vi "channelGraphs.vi"(8 "error in (no error)":errorcluster, 10 "Clean+No Dups":string[][](array[string])) -> (0 "error out":errorcluster, 1 "Noisy Pixel List":i32[][](array[numeric]), 2 "Intensity Graph":u32[][](graph), 3 "Detector Surface":refnum<class "3D Plot Datatype.lvclass">[](xcontrol), 5 "Event Count Histogram":T1(graph))   [LabVIEW 2019]
uses:
  <vilib>/Analysis/NI_AALBase.lvlib
  <vilib>/Math Plots/3D Math Plots/3D Surface/3D Surface Datatype/3D Surface Datatype.lvclass
  <vilib>/Math Plots/3D Math Plots/3D Surface/3D Surface Datatype/Public/Plot Helper (Vector).vi
  <vilib>/Math Plots/3D Math Plots/3D Surface/3D Surface XCtrl/3D Surface.xctl
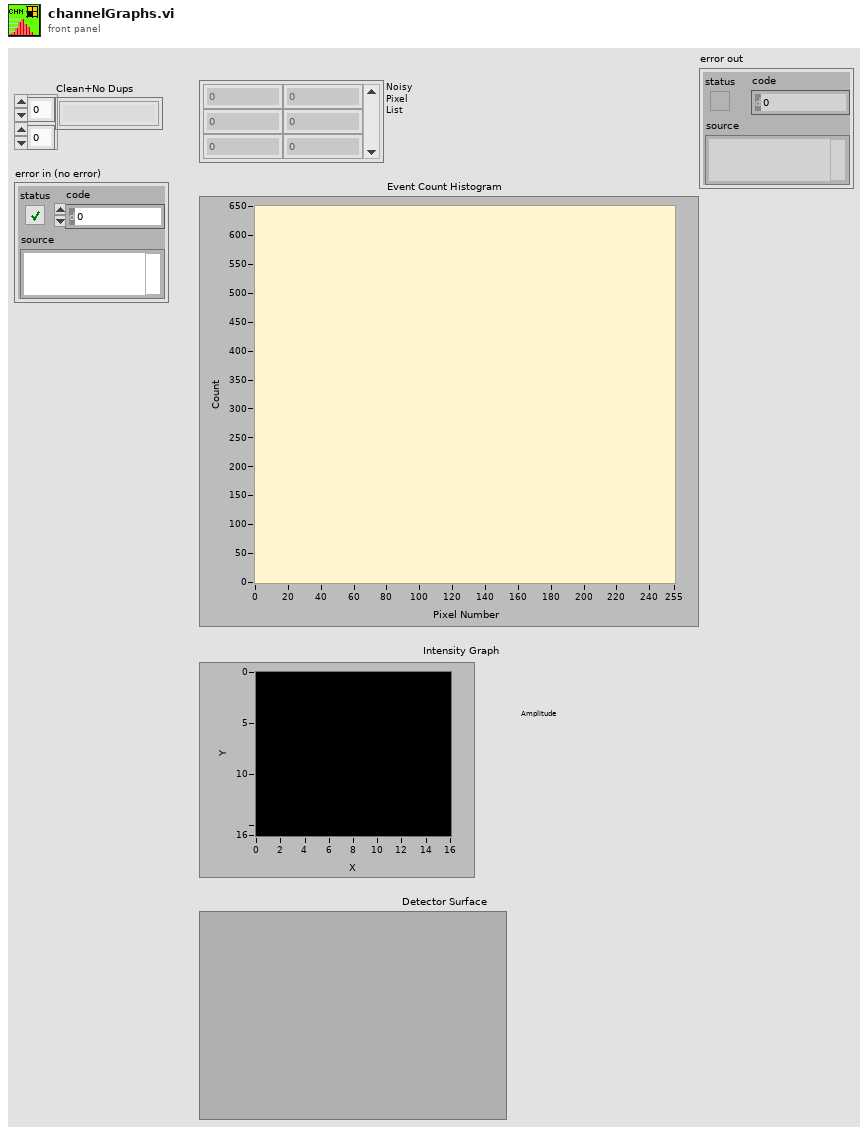
[diagram p1: front panel]
types:
  T1 = cluster{"X Values":dbl[], "Histogram: h(x)":i32[]}
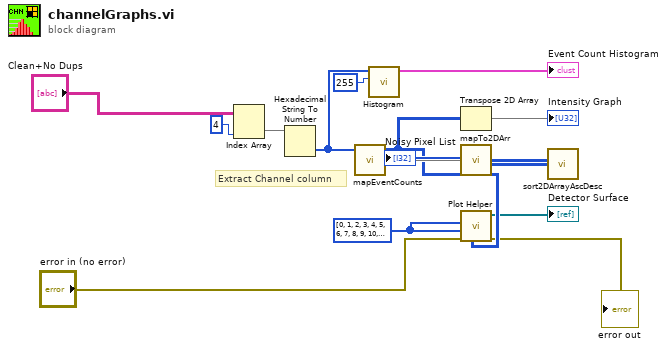
[diagram p0: block diagram]
diagram:
  w15 = u8[] [0, 1, 2, 3, 4, 5, 6, 7, 8, 9, 10, 11, 12, 13, 14, 15, 0, 1, 2, 3, 4, 5, 6, 7, 8, 9, 10, 11, 12, 13, 14, 15, 0, 1, 2, 3, 4, 5, 6, 7, 8, 9, 10, 11, 12, 13, 14, 15, 0, 1, 2, 3, 4, 5, 6, 7, 8, 9, 10, 11, 12, 13, 14, 15, 0, 1, 2, 3, 4, 5, 6, 7, 8, 9, 10, 11, 12, 13, 14, 15, 0, 1, 2, 3, 4, 5, 6, 7, 8, 9, 10, 11, 12, 13, 14, 15, 0, 1, 2, 3, 4, 5, 6, 7, 8, 9, 10, 11, 12, 13, 14, 15, 0, 1, 2, 3, 4, 5, 6, 7, 8, 9, 10, 11, 12, 13, 14, 15, 0, 1, 2, 3, 4, 5, 6, 7, 8, 9, 10, 11, 12, 13, 14, 15, 0, 1, 2, 3, 4, 5, 6, 7, 8, 9, 10, 11, 12, 13, 14, 15, 0, 1, 2, 3, 4, 5, 6, 7, 8, 9, 10, 11, 12, 13, 14, 15, 0, 1, 2, 3, 4, 5, 6, 7, 8, 9, 10, 11, 12, 13, 14, 15, 0, 1, 2, 3, 4, 5, 6, 7, 8, 9, 10, 11, 12, 13, 14, 15, 0, 1, 2, 3, 4, 5, 6, 7, 8, 9, 10, 11, 12, 13, 14, 15, 0, 1, 2, 3, 4, 5, 6, 7, 8, 9, 10, 11, 12, 13, 14, 15, 0, 1, 2, 3, 4, 5, 6, 7, 8, 9, 10, 11, 12, 13, 14] ("Array")
  # "Extract Channel column"
  n1 = Index Array(array="Clean+No Dups", index (col)=4 ("disabled index (col)")) -> (element=w13:string[])  [unwired: 1 in]
  n2 = Hexadecimal String To Number(string=w13) -> (number=w14:u32[])  [unwired: 2 in, 1 out]
  n3 = call "mapEventCounts.vi"("Count"=w14) -> ("Counts (map)"=w11:map{u32, u32}, "Count Grid"=w7:u32[][])  [unwired: 3 in]
  n4 = call <vilib>:"Histogram.vi"("intervals"=255, "X"=w14) -> ("Histogram Graph"=→"Event Count Histogram":T1)  [unwired: 5 in, 4 out]
  n5 = Transpose 2D Array(2D array=w7) -> (transposed array=→"Intensity Graph":u32[][])
  n6 = call "mapTo2DArr.vi"("Map"=w11) -> ("2D Array"=w10:i32[][])
  n7 = call-poly <vilib>:"Plot Helper.vi"("z matrix"=w7, "error in (no error)"="error in (no error)", "y vector"=w15, "x vector"=w15) -> ("error out"=→"error out":errorcluster, "3D Plot lvclass Array out"=→"Detector Surface":refnum<class "3D Plot Datatype.lvclass">[])  [unwired: 2 in, 4 out]
  n8 = call "sort2DArrayAscDesc.vi"("2D Array"=w10) -> ("sorted 2D array"=→"Noisy Pixel List":i32[][])  [unwired: 5 in]
